vi "Get Column Factory.vi"(8 "error in (no error)":errorcluster, 11 "Table Configuration in":refnum<class "Table Configuration.lvclass">) -> (0 "error out":errorcluster, 2 "Column Factory":refnum<class "Column Factory.lvclass">, 3 "Table Configuration out":refnum<class "Table Configuration.lvclass">)   [LabVIEW 2020, in "Table.lvlib" / "Table Configuration.lvclass"]
uses:
  Table Configuration.lvclass
  Column Factory/Column Factory.lvclass
  Table Configuration.lvclass/Table Configuration.ctl
  Basic Column Factory/Basic Column Factory.lvclass
  C:/Users/User/Desktop/Raman Program/Database OOP/source/Database OOP/Column Factory/Column Factory.lvclass
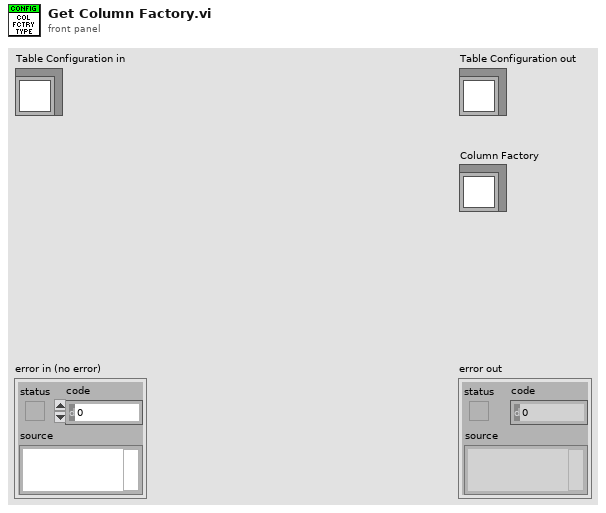
[diagram p1: front panel]
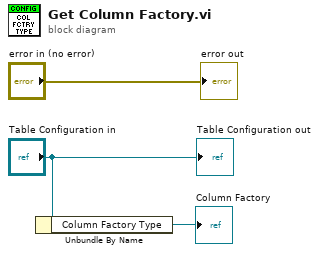
[diagram p0: block diagram]
diagram:
  n1 = Unbundle By Name("Table Configuration in") -> ("Column Factory Type"=→"Column Factory":refnum<class "Basic Column Factory.lvclass">)
  "error out" <- "error in (no error)"
  "Table Configuration out" <- "Table Configuration in"
